vi "test_RS-xxx Read With Termination Character.vi"(8 "error in (no error)":errorcluster, 11 "TestCase in":refnum<class "Instrument Addon Serial Protocols Unit Tests.lvclass">) -> (0 "error out":errorcluster, 3 "TestCase out":refnum<class "Instrument Addon Serial Protocols Unit Tests.lvclass">)   [LabVIEW 2023, in "Instrument Addon Serial Protocols Unit Tests.lvclass"]
uses:
  Instrument Addon Serial Protocols Unit Tests.lvclass
  Instrument Addon Serial Protocols Unit Tests.lvclass/Instrument Addon Serial Protocols Unit Tests.ctl
  <vilib>/addons/_JKI Toolkits/VI Tester/TestCase.llb/TestCase.lvclass
  Listener/Listener.lvclass
  Listener/ListenerClassControls/Operation.ctl
  <vilib>/platform/TimedLoop/XDataNode/XDataNode.xnode
  <vilib>/Platform/TimedLoop/XDataNode/nitl_modes.ctl
  <vilib>/Platform/TimedLoop/XDataNode/XDNodeRunTimeDep.lvlib
  <vilib>/Platform/TimedLoop/XDataNode/wakeup.ctl
  <vilib>/Platform/TimedLoop/XDataNode/timing_clust.ctl
  RS-xxx/RS-xxx.lvclass
  Protocol Parent/Methods/Read Parameter.ctl
  Protocol Parent/Protocol Parent.lvclass
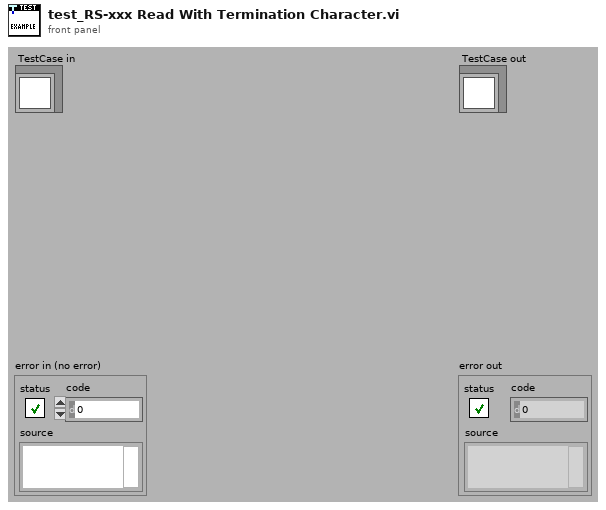
[diagram p1: front panel]
types:
  T1 = typedef "Protocols.lvlib/Protocol Parent.lvclass/Read Parameter.ctl" = cluster{"Wait Type":enum16{"Byte Count", "Wait sec"}, "Wait Value":dbl}
  T2 = typedef "Listener.lvclass/Operation.ctl" = enum16{"Read", "Write"}
  T3 = typedef "XDNodeRunTimeDep.lvlib/timing_clust.ctl" = cluster{"Expected End [f-1]":u64, "Actual End [f-1]":u64, "Finished Late? [f-1]":bool, "Expected End [i-1]":u64, "Actual End [i-1]":u64, "Finished Late? [i-1]":bool, "Expected Start [i]":u64, "Actual Start [i]":u64, "Expected Start [f]":u64, "Actual Start [f]":u64, "Source Name":string, "Structure Name":string, "Period":i64, "Deadline":i64, "Offset":i64, "Start":i64, "Priority":i32, "Timeout":i32, "Mode":T4, "Wakeup Reason":T5, "Error":errorcluster, "Source Type":string, "Secondary Source Type":string, "Global End Time":u64, "Global Start Time":u64, "Frame Duration":u64, "Iteration Duration":u64, "Assigned CPU":i32, "I/O Scan Engine Mode":u32}
  T4 = typedef "XDNodeRunTimeDep.lvlib/nitl_modes.ctl" = enum32{"No Change", "Process missed periods, maintain original phase", "Discard missed periods, maintain original phase", "Process missed periods, ignore original phase", "Discard missed periods, ignore original phase"}
  T5 = typedef "XDNodeRunTimeDep.lvlib/wakeup.ctl" = enum32{"Normal", "Aborted", "Asynchronous wakeup", "Timing source error", "Timed loop error", "Timeout"}
  T6 = typedef "Listener.lvclass/RS-xxx Data Structure.ctl" = cluster{"Virtual COM Port Settings 1":cluster{"Port":string, "Baud Rate":u32, "Data Bits":u16, "Parity":enum16{"None", "Odd", "Even", "Mark", "Space"}, "Stop Bits":u16, "Flow Control":u16, "XON":enum16{"NUL", "SOH", "STX", "ETX", "EOT", "ENQ", "ACK", "BEL", "BS", "HT", "LF", "VT", "FF", "CR", "SO", "SI", "DLE", "DC1", "DC2", "DC3", "DC4", "NAK", "SYN", "ETB", "CAN", "EM", "SUB", "ESC", "FS", "GS", "RS", "US", "SP", "!", "\"", "#", "$", "%", "&", "'", "(", ")", "*", "+", ",", "- (-)", ".", "/", "0", "1", "2", "3", "4", "5", "6", "7", "8", "9", ":", ";", "<", "=", ">", "?", "@", "A", "B", "C", "D", "E", "F", "G", "H", "I", "J", "K", "L", "M", "N", "O", "P", "Q", "R", "S", "T", "U", "V", "W", "X", "Y", "Z", "[", "\\", "]", "^", "_", "`", "a", "b", "c", "d", "e", "f", "g", "h", "i", "j", "k", "l", "m", "n", "o", "p", "q", "r", "s", "t", "u", "v", "w", "x", "y", "z", "{", "|", "}", "~"}, "XOFF":enum16{"NUL", "SOH", "STX", "ETX", "EOT", "ENQ", "ACK", "BEL", "BS", "HT", "LF", "VT", "FF", "CR", "SO", "SI", "DLE", "DC1", "DC2", "DC3", "DC4", "NAK", "SYN", "ETB", "CAN", "EM", "SUB", "ESC", "FS", "GS", "RS", "US", "SP", "!", "\"", "#", "$", "%", "&", "'", "(", ")", "*", "+", ",", "- (-)", ".", "/", "0", "1", "2", "3", "4", "5", "6", "7", "8", "9", ":", ";", "<", "=", ">", "?", "@", "A", "B", "C", "D", "E", "F", "G", "H", "I", "J", "K", "L", "M", "N", "O", "P", "Q", "R", "S", "T", "U", "V", "W", "X", "Y", "Z", "[", "\\", "]", "^", "_", "`", "a", "b", "c", "d", "e", "f", "g", "h", "i", "j", "k", "l", "m", "n", "o", "p", "q", "r", "s", "t", "u", "v", "w", "x", "y", "z", "{", "|", "}", "~"}, "End Read on Termination Character":bool, "End Write on Termination Character":bool, "Termination Character":u8}, "Virtual COM Port Settings 2":cluster{"Port":string, "Baud Rate":u32, "Data Bits":u16, "Parity":enum16{"None", "Odd", "Even", "Mark", "Space"}, "Stop Bits":u16, "Flow Control":u16, "XON":enum16{"NUL", "SOH", "STX", "ETX", "EOT", "ENQ", "ACK", "BEL", "BS", "HT", "LF", "VT", "FF", "CR", "SO", "SI", "DLE", "DC1", "DC2", "DC3", "DC4", "NAK", "SYN", "ETB", "CAN", "EM", "SUB", "ESC", "FS", "GS", "RS", "US", "SP", "!", "\"", "#", "$", "%", "&", "'", "(", ")", "*", "+", ",", "- (-)", ".", "/", "0", "1", "2", "3", "4", "5", "6", "7", "8", "9", ":", ";", "<", "=", ">", "?", "@", "A", "B", "C", "D", "E", "F", "G", "H", "I", "J", "K", "L", "M", "N", "O", "P", "Q", "R", "S", "T", "U", "V", "W", "X", "Y", "Z", "[", "\\", "]", "^", "_", "`", "a", "b", "c", "d", "e", "f", "g", "h", "i", "j", "k", "l", "m", "n", "o", "p", "q", "r", "s", "t", "u", "v", "w", "x", "y", "z", "{", "|", "}", "~"}, "XOFF":enum16{"NUL", "SOH", "STX", "ETX", "EOT", "ENQ", "ACK", "BEL", "BS", "HT", "LF", "VT", "FF", "CR", "SO", "SI", "DLE", "DC1", "DC2", "DC3", "DC4", "NAK", "SYN", "ETB", "CAN", "EM", "SUB", "ESC", "FS", "GS", "RS", "US", "SP", "!", "\"", "#", "$", "%", "&", "'", "(", ")", "*", "+", ",", "- (-)", ".", "/", "0", "1", "2", "3", "4", "5", "6", "7", "8", "9", ":", ";", "<", "=", ">", "?", "@", "A", "B", "C", "D", "E", "F", "G", "H", "I", "J", "K", "L", "M", "N", "O", "P", "Q", "R", "S", "T", "U", "V", "W", "X", "Y", "Z", "[", "\\", "]", "^", "_", "`", "a", "b", "c", "d", "e", "f", "g", "h", "i", "j", "k", "l", "m", "n", "o", "p", "q", "r", "s", "t", "u", "v", "w", "x", "y", "z", "{", "|", "}", "~"}, "End Read on Termination Character":bool, "End Write on Termination Character":bool, "Termination Character":u8}, "Data":string, "Data Length":u32}
  T7 = cluster{"Port":string, "Baud Rate":u32, "Data Bits":u16, "Parity":enum16{"None", "Odd", "Even", "Mark", "Space"}, "Stop Bits":u16, "Flow Control":u16, "XON":enum16{"NUL", "SOH", "STX", "ETX", "EOT", "ENQ", "ACK", "BEL", "BS", "HT", "LF", "VT", "FF", "CR", "SO", "SI", "DLE", "DC1", "DC2", "DC3", "DC4", "NAK", "SYN", "ETB", "CAN", "EM", "SUB", "ESC", "FS", "GS", "RS", "US", "SP", "!", "\"", "#", "$", "%", "&", "'", "(", ")", "*", "+", ",", "- (-)", ".", "/", "0", "1", "2", "3", "4", "5", "6", "7", "8", "9", ":", ";", "<", "=", ">", "?", "@", "A", "B", "C", "D", "E", "F", "G", "H", "I", "J", "K", "L", "M", "N", "O", "P", "Q", "R", "S", "T", "U", "V", "W", "X", "Y", "Z", "[", "\\", "]", "^", "_", "`", "a", "b", "c", "d", "e", "f", "g", "h", "i", "j", "k", "l", "m", "n", "o", "p", "q", "r", "s", "t", "u", "v", "w", "x", "y", "z", "{", "|", "}", "~"}, "XOFF":enum16{"NUL", "SOH", "STX", "ETX", "EOT", "ENQ", "ACK", "BEL", "BS", "HT", "LF", "VT", "FF", "CR", "SO", "SI", "DLE", "DC1", "DC2", "DC3", "DC4", "NAK", "SYN", "ETB", "CAN", "EM", "SUB", "ESC", "FS", "GS", "RS", "US", "SP", "!", "\"", "#", "$", "%", "&", "'", "(", ")", "*", "+", ",", "- (-)", ".", "/", "0", "1", "2", "3", "4", "5", "6", "7", "8", "9", ":", ";", "<", "=", ">", "?", "@", "A", "B", "C", "D", "E", "F", "G", "H", "I", "J", "K", "L", "M", "N", "O", "P", "Q", "R", "S", "T", "U", "V", "W", "X", "Y", "Z", "[", "\\", "]", "^", "_", "`", "a", "b", "c", "d", "e", "f", "g", "h", "i", "j", "k", "l", "m", "n", "o", "p", "q", "r", "s", "t", "u", "v", "w", "x", "y", "z", "{", "|", "}", "~"}, "End Read on Termination Character":bool, "End Write on Termination Character":bool, "Termination Character":u8}
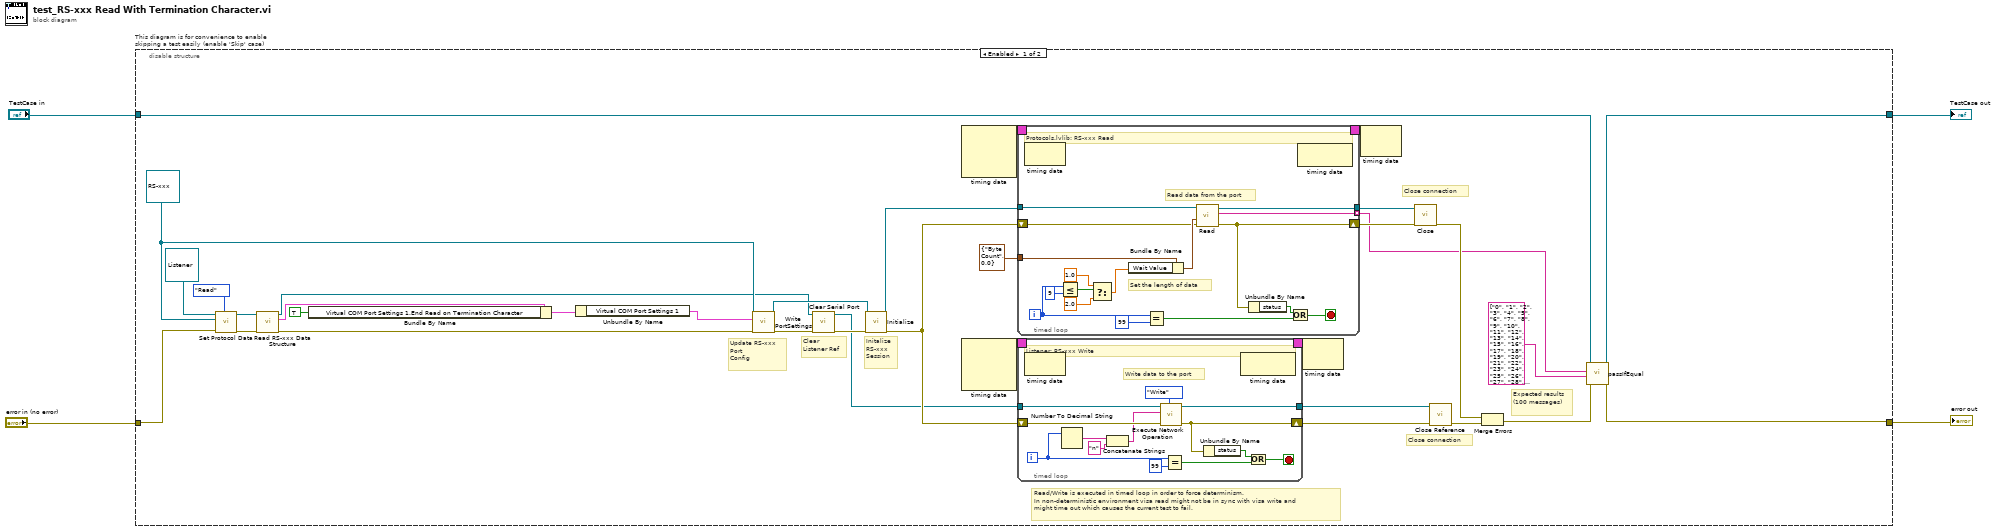
[diagram p0: block diagram]
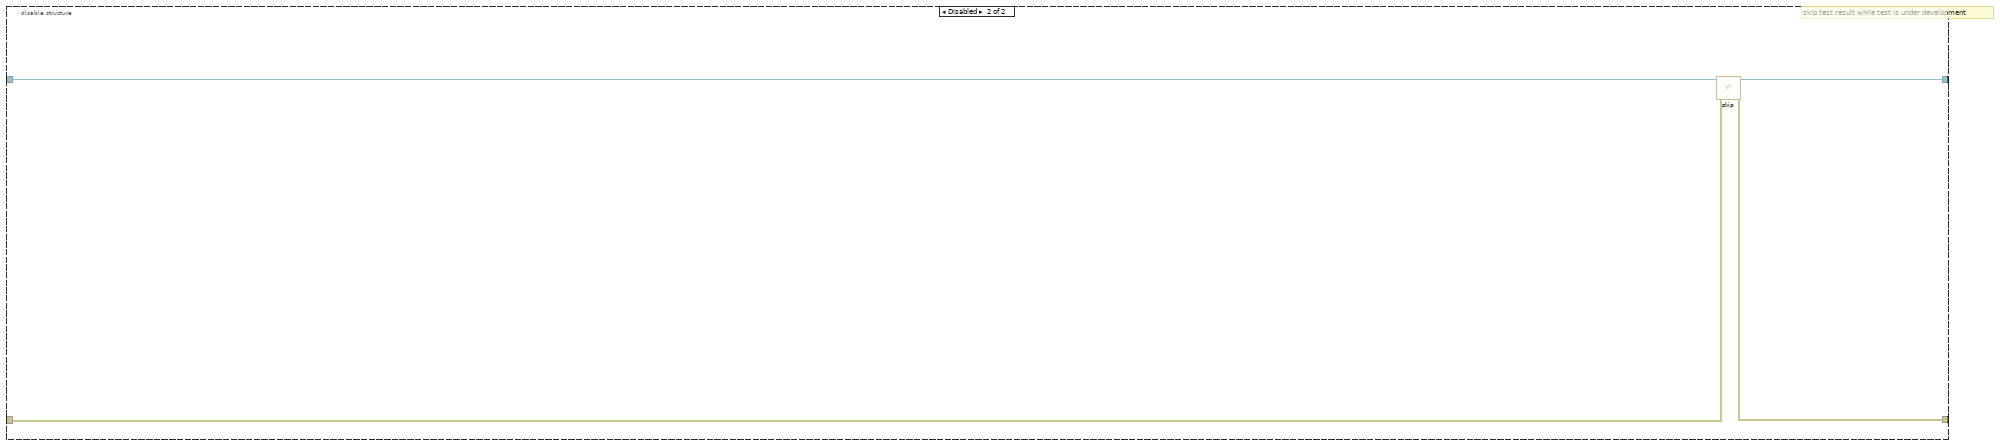
[diagram p2: hidden frame]
diagram:
  n1 = disable-structure "This diagram is for convenience to enable skipping a test easily (enable 'Skip' case)" shown="Enabled" {
    disable-tunnel: "TestCase in" -> [w39 w81]
    disable-tunnel: [w38 w79] -> w2
    disable-tunnel: [w37 w80] -> w4
    disable-tunnel: "error in (no error)" -> [w33 w78]
    frame Enabled {
      w21 = refnum<class "RS-xxx.lvclass"> refnum ("Protocols.lvlib:RS-xxx.lvclass")
      # "Clear \nListener Ref"
      # "Update RS-xxx \nPort \nConfig"
      # "Initalize \nRS-xxx\nSession"
      # "Close connection"
      # "Close connection"
      # "Read/Write is executed in timed loop in order to force determinism.\nIn non-deterministic environment visa read might not be in sync with visa write and\nmight time out which causes the current test to fail."
      # "Expected results\n(100 messages)"
      n2 = call "Set Protocol Data.vi"("Operation"=Operation."Read", "error in (no error)"=w33, "Protocols.lvlib:Protocol Parent.lvclass"=w21, "Listener In.lvclass"=refnum<class "Listener.lvclass"> refnum ("Listener.lvclass")) -> ("error out"=w22:errorcluster, "Listener Out.lvclass"=w23:refnum<class "Listener.lvclass">)  [unwired: 6 in]
      n3 = call-dynamic "Read RS-xxx Data Structure.vi"("error in (no error)"=w22, "Listener in"=w23) -> ("error out"=w6:errorcluster, "RS-xxx Data Structure"=w10:T6, "Listener out"=w5:refnum<class "Listener.lvclass">)  [unwired: 7 in]
      n4 = Bundle By Name(cluster=w10, "Virtual COM Port Settings 1.End Read on Termination Character"=TRUE) -> (w8:T6)
      n5 = Unbundle By Name(w8) -> ("Virtual COM Port Settings 1"=w7:T7)
      n6 = call "Write PortSettings.vi"("error in (no error)"=w6, "PortSettings"=w7, "RS232 in"=w21) -> ("error out"=w15:errorcluster, "RS232 out"=w20:refnum<class "RS-xxx.lvclass">)  [unwired: 7 in]
      n7 = call "Clear Serial Port.vi"("error in (no error)"=w15, "Listener In.lvclass"=w5) -> ("error out"=w14:errorcluster, "Listener out"=w11:refnum<class "Listener.lvclass">)  [unwired: 8 in]
      n8 = call-dynamic "Initialize.vi"("error in (no error)"=w14, "RS232 in"=w20) -> ("error out"=w13:errorcluster, "RS232 out"=w19:refnum<class "RS-xxx.lvclass">)  [unwired: 8 in]
      n9 = node-c288() -> (w27:T3)  [unwired: 3 in]
      n10 = node-c288() -> (w25:T3)  [unwired: 3 in]
      n11 = timed-loop {
        shift-right: [w60] -> w30
        shift-left: w13 -> [w57]
        timing: w27 -> [_]
        timing-out: [_] -> w26
        tunnel: w19 -> [w58]
        tunnel: T1 {"Wait Type"=enum."Byte Count", "Wait Value"=0.0} ("Read Parameter") -> [w70]
        tunnel: [w68] -> w17
        tunnel: [w67] -> w16 mode=indexing
        i -> [w66]
        stop <- w71 stop-if-true
        # "Set the length of data"
        # "Read data from the port"
        # "Protocols.lvlib: RS-xxx Read"
        n12 = node-c288() -> ()  [unwired: 1 in, 1 out]
        n13 = Less Or Equal?(x=w66, y=9) -> (x <= y?=w64:bool)
        n14 = Select(t=1.0, s=w64, f=2.0) -> (s? t:f=w61:dbl)
        n15 = Bundle By Name(cluster=w70, "Wait Value"=w61) -> (w69:T1)
        n16 = Equal?(x=w66, y=99) -> (x = y?=w73:bool)
        n17 = call-dynamic "Read.vi"("error in (no error)"=w57, "Variant"=w69, "RS232 in"=w58) -> ("error out"=w60:errorcluster, "String"=w67:string, "RS232 out"=w68:refnum<class "RS-xxx.lvclass">)  [unwired: 6 in]
        n18 = Unbundle By Name(w60) -> ("status"=w59:bool)
        n19 = Or(x=w59, y=w73) -> (x .or. y?=w71:bool)
        n20 = node-c288() -> ()  [unwired: 1 in, 1 out]
      }
      n21 = timed-loop {
        shift-right: [w44] -> w28
        shift-left: w13 -> [w46]
        tunnel: [w48] -> w29
        timing: w25 -> [_]
        timing-out: [_] -> w24
        tunnel: w11 -> [w47]
        i -> [w45]
        stop <- w49 stop-if-true
        # "Write data to the port"
        # "Listener: RS-xxx Write"
        n22 = node-c288() -> ()  [unwired: 1 in, 1 out]
        n23 = Number To Decimal String(number=w45) -> (decimal integer string=w42:string)  [unwired: 1 in]
        n24 = Concatenate Strings(w42, "n" ("string")) -> (w40:string)
        n25 = call "Execute Network Operation.vi"("Operation"=Operation."Write", "error in (no error)"=w46, "Message"=w40, "Listener In.lvclass"=w47) -> ("error out"=w44:errorcluster, "Listener Out.lvclass"=w48:refnum<class "Listener.lvclass">)  [unwired: 6 in]
        n26 = Equal?(x=w45, y=99) -> (x = y?=w50:bool)
        n27 = Unbundle By Name(w44) -> ("status"=w43:bool)
        n28 = node-c288() -> ()  [unwired: 1 in, 1 out]
        n29 = Or(x=w43, y=w50) -> (x .or. y?=w49:bool)
      }
      n30 = node-c288(w24) -> ()  [unwired: 1 out]
      n31 = node-c288(w26) -> ()  [unwired: 1 out]
      n32 = call-dynamic "Close.vi"("error in (no error)"=w30, "RS232 in"=w17) -> ("error out"=w32:errorcluster)  [unwired: 8 in, 1 out]
      n33 = call "Close Reference.vi"("error in (no error)"=w28, "Listener In.lvclass"=w29) -> ("error out"=w31:errorcluster)  [unwired: 8 in, 1 out]
      n34 = Merge Errors(w32, w31) -> (w34:errorcluster)
      n35 = call-dynamic "passIfEqual.vi"("error in (no error)"=w34, "y"=string[] ["0", "1", "2", "3", "4", "5", "6", "7", "8", "9", "10", "11", "12", "13", "14", "15", "16", "17", "18", "19", "20", "21", "22", "23", "24", "25", "26", "27", "28", "29", "30", "31", "32", "33", "34", "35", "36", "37", "38", "39", "40", "41", "42", "43", "44", "45", "46", "47", "48", "49", "50", "51", "52", "53", "54", "55", "56", "57", "58", "59", "60", "61", "62", "63", "64", "65", "66", "67", "68", "69", "70", "71", "72", "73", "74", "75", "76", "77", "78", "79", "80", "81", "82", "83", "84", "85", "86", "87", "88", "89", "90", "91", "92", "93", "94", "95", "96", "97", "98", "99"] ("Array"), "x"=w16, "TestCase in"=w39) -> ("error out"=w37:errorcluster, "TestCase out"=w38:refnum<class "Instrument Addon Serial Protocols Unit Tests.lvclass">)  [unwired: 6 in]
    }
    frame Disabled {
      # "skip test result while test is under development"
      n36 = call <vilib>:"skip.vi"("error in (no error)"=w78, "TestCase in"=w81) -> ("error out"=w80:errorcluster, "TestCase out"=w79:refnum<class "Instrument Addon Serial Protocols Unit Tests.lvclass">)  [unwired: 8 in]
    }
  }
  "error out" <- w4
  "TestCase out" <- w2
